vi "LWXPS_GroupJogParametersGet.vi"(8 "LabVIEW error IN":errorcluster, 9 "Number of positioners":i32, 10 "Group Name":string, 11 "XPS Reference IN":refnum<k24>) -> (0 "XPS Error String":string, 1 "Acceleration":dbl[](array[numeric]), 2 "Velocity":dbl[](array[numeric]), 3 "Returned error code":i32, 4 "LabVIEW error OUT":errorcluster, 5 "XPS Reference OUT":refnum<k24>)   [LabVIEW 2014]
uses:
  D:/XPSQ8_LabView_Library/Development/Source/Dll/Newport.XPS.CommandInterface.dll
  Dll/Newport.XPS.CommandInterface.dll
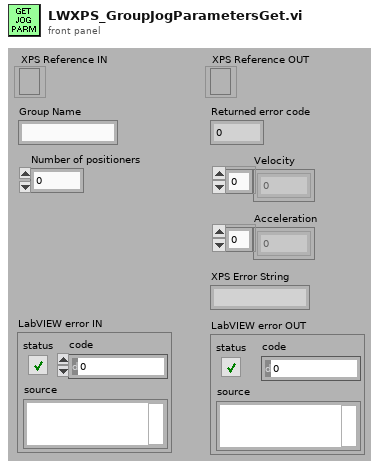
[diagram p1: front panel]
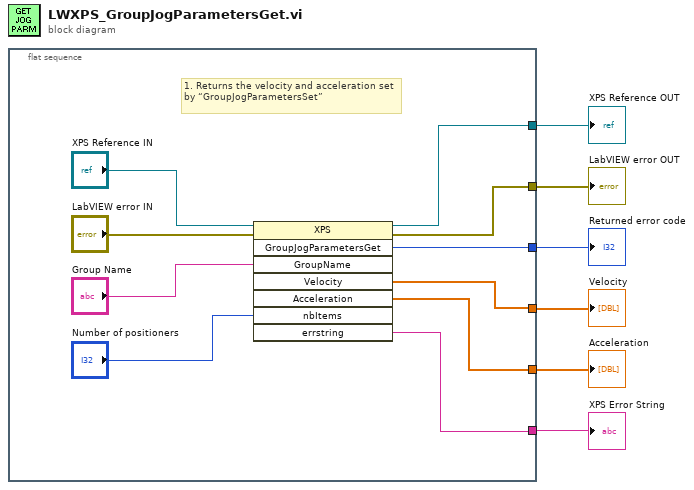
[diagram p0: block diagram]
diagram:
  n1 = flat-sequence {
    tunnel: [w8] -> w6
    tunnel: [w13] -> w5
    tunnel: [w15] -> w4
    tunnel: [w12] -> w2
    tunnel: [w7] -> w1
    tunnel: [w9] -> w3
    frame #0 {
      # "1. Returns the velocity and acceleration set by “GroupJogParametersSet”"
      n2 = invoke class="XPS" method="GroupJogParametersGet"(reference="XPS Reference IN", error in="LabVIEW error IN", "GroupName"="Group Name", "nbItems"="Number of positioners") -> (reference out=w8:refnum<k24>, error out=w13:errorcluster, "GroupJogParametersGet"=w15:i32, "Velocity"=w9:dbl[], "Acceleration"=w12:dbl[], "errstring"=w7:string)  [unwired: 4 in, 2 out]
    }
  }
  "XPS Reference OUT" <- w6
  "LabVIEW error OUT" <- w5
  "Returned error code" <- w4
  "XPS Error String" <- w1
  "Velocity" <- w3
  "Acceleration" <- w2
